vi "CorrecionMicrofono.vi"(3 "row in":i32, 4 "Medido":dbl, 5 "Prueba031 in":refnum<class "Prueba03.lvclass">) -> (0 "row out":i32, 1 "Medido Corregido":dbl, 2 "Prueba031 out":refnum<class "Prueba03.lvclass">)   [LabVIEW 2019, in "Prueba03.lvclass"]
uses:
  Prueba03.lvclass
  Prueba03.lvclass/Prueba03.ctl
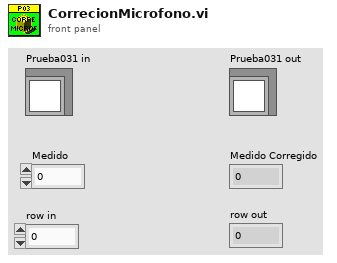
[diagram p1: front panel]
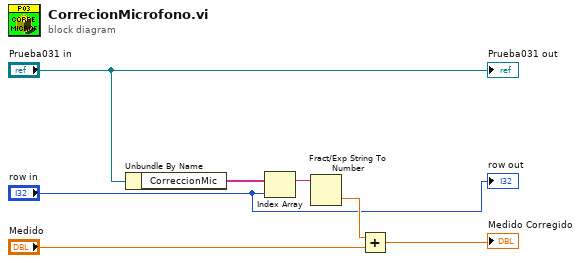
[diagram p0: block diagram]
diagram:
  n1 = Unbundle By Name("Prueba031 in") -> ("CorreccionMic"=w6:string[])
  n2 = Index Array(array=w6, index="row in") -> (element=w2:string)
  n3 = Fract/Exp String To Number(string=w2) -> (number=w3:dbl)  [unwired: 3 in, 1 out]
  n4 = Add(x=w3, y="Medido") -> (x+y=→"Medido Corregido":dbl)
  "Prueba031 out" <- "Prueba031 in"
  "row out" <- "row in"
